vi "Init.vi"(8 "error in (no error)":errorcluster, 10 "VISA resource name":refnum<visa-resource-name>, 11 "Reload-pro in":refnum<class "Reload-pro.lvclass">) -> (0 "error out":errorcluster, 3 "Reload-pro out":refnum<class "Reload-pro.lvclass">)   [LabVIEW 2013, in "Reload-pro.lvclass"]
uses:
  Reload-pro.lvclass
  Reload-pro.lvclass/Reload-pro.ctl
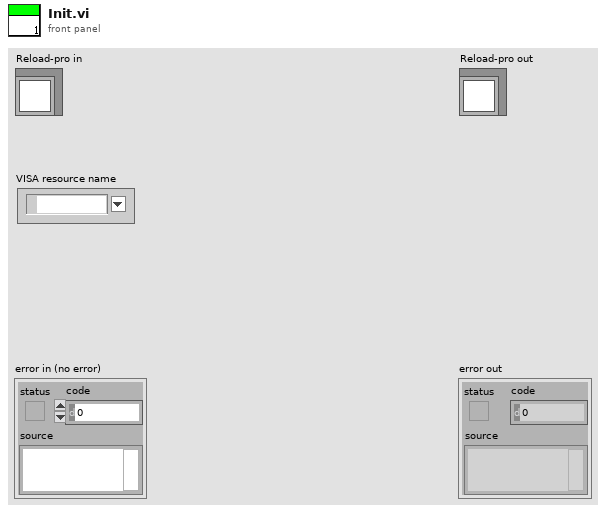
[diagram p1: front panel]
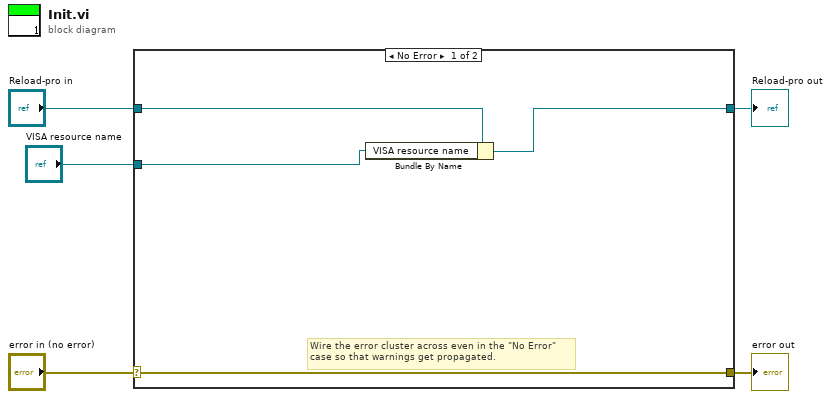
[diagram p0: block diagram]
diagram:
  n1 = case shown="No Error" "error in (no error)" {
    selector: "error in (no error)" -> [w9 w11]
    tunnel: [w9 w11] -> w4
    tunnel: [w7 w10] -> w2
    tunnel: "Reload-pro in" -> [w8 w10]
    tunnel: "VISA resource name" -> [w6 _]
    frame No Error {
      # "Wire the error cluster across even in the \"No Error\"\ncase so that warnings get propagated."
      n2 = Bundle By Name(cluster=w8, "VISA resource name"=w6) -> (w7:refnum<class "Reload-pro.lvclass">)
    }
    frame Error {
    }
  }
  "error out" <- w4
  "Reload-pro out" <- w2
